vi "closeHandler.vi"(8 "error in (no error)":errorcluster, 11 "Handler.File in":refnum<class "Handler.File.lvclass">) -> (0 "error out":errorcluster, 3 "Handler.File out":refnum<class "Handler.File.lvclass">)   [LabVIEW 2017, in "Error Log.lvlib" / "Handler.File.lvclass"]
uses:
  Handler.File.lvclass
  Handler/Handler.lvclass
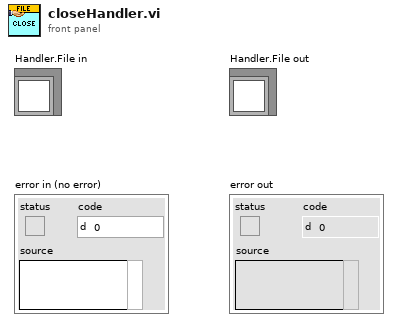
[diagram p1: front panel]
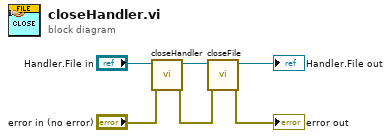
[diagram p0: block diagram]
diagram:
  n1 = call-parent "closeHandler.vi"("error in (no error)"="error in (no error)", "Handler in"="Handler.File in") -> ("error out"=w2:errorcluster, "Handler out"=w6:refnum<class "Handler.File.lvclass">)  [unwired: 8 in]
  n2 = call-dynamic "closeFile.vi"("error in (no error)"=w2, "Handler.File in"=w6) -> ("error out"=→"error out":errorcluster, "Handler.File out"=→"Handler.File out":refnum<class "Handler.File.lvclass">)  [unwired: 8 in]
